vi "Print.vi"(8 "error in (no error)":errorcluster, 11 "reference in":refnum<class "PrintVisitor.lvclass">) -> (0 "error out":errorcluster, 2 "Id String":string, 3 "reference in":refnum<class "PrintVisitor.lvclass">)   [LabVIEW 2020, in "PrintVisitor.lvclass"]
uses:
  PrintVisitor.lvclass
  Equipment_class/Equipment.lvclass
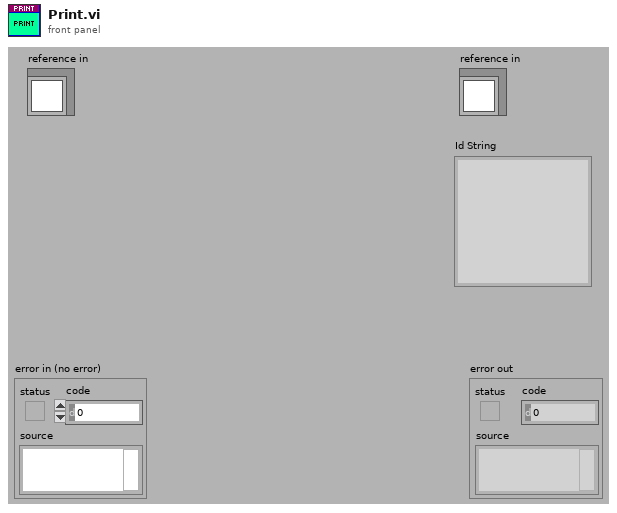
[diagram p1: front panel]
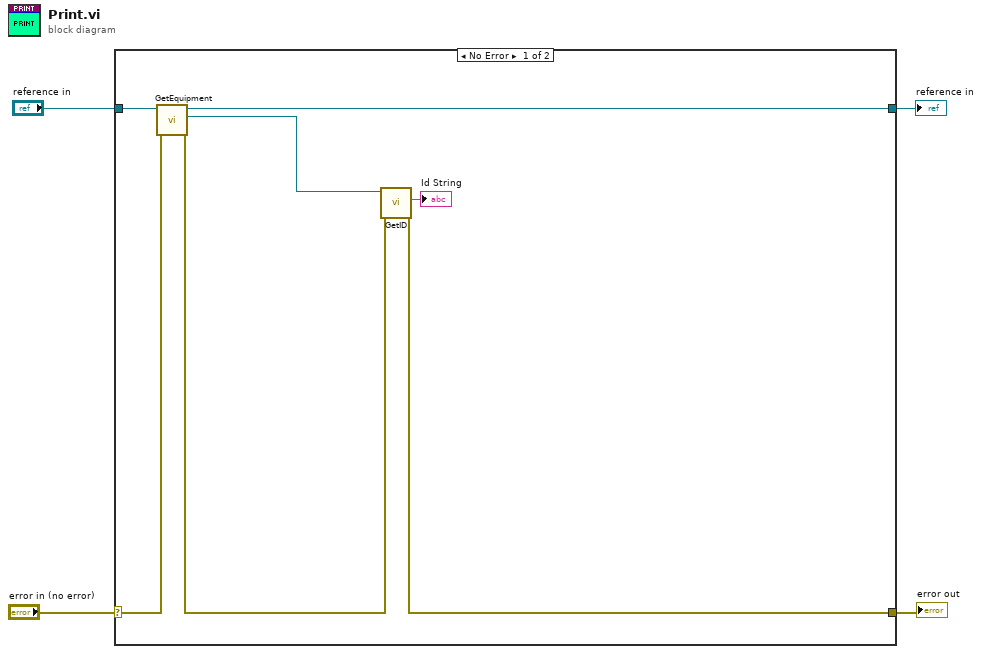
[diagram p0: block diagram]
diagram:
  n1 = case shown="No Error" "error in (no error)" {
    selector: "error in (no error)" -> [w10 w13]
    tunnel: [w6 w13] -> w3
    tunnel: [w9 w12] -> w1
    tunnel: "reference in" -> [w11 w12]
    frame No Error {
      n2 = call-dynamic "GetEquipment.vi"("error in (no error)"=w10, "reference in"=w11) -> ("error out"=w7:errorcluster, "Equipment"=w8:refnum<class "Equipment.lvclass">, "reference out"=w9:refnum<class "PrintVisitor.lvclass">)  [unwired: 7 in]
      n3 = call-dynamic "GetID.vi"("error in (no error)"=w7, "reference in"=w8) -> ("error out"=w6:errorcluster, "Id String"=→"Id String":string)  [unwired: 7 in, 1 out]
    }
    frame Error {
    }
  }
  "error out" <- w3
  "reference in" <- w1
